vi "Write VISA Commands.vi"(6 "CMD Prefix":string, 7 "CMDs":string[](array[string]), 8 "error in":errorcluster, 9 "<JSON> Object":string, 10 "JSON Keys":string[](array[string]), 11 "VISA Refnum in":refnum<visa-resource-name>) -> (0 "error out":errorcluster, 3 "VISA Refnum out":refnum<visa-resource-name>)   [LabVIEW 2023, in "Continuous Waveform Acq CFG.lvclass"]
uses:
  Continuous Waveform Acq CFG.lvclass
  98ddc1df-d889-4f20-b281-f2799059f154.vi
  <vilib>/JDP Science/JSONtext/Find Item.vi
  <vilib>/JDP Science/JSONtext/Next JSON Value.vi
  <vilib>/JDP Science/JSONtext/String Subset.vi
  <vilib>/JDP Science/JSONtext/Parsing/Advance past next JSON Value (inlined COPY).vi
  <vilib>/JDP Science/JSONtext/Parsing/Advance past whitespace.vi
  <vilib>/JDP Science/JSONtext/Parsing/Advance past String.vi
  <vilib>/JDP Science/JSONtext/Parsing/Advance past Number.vi
  <vilib>/JDP Science/JSONtext/Parsing/Advance past Line Ending.vi
  <vilib>/JDP Science/JSONtext/Parsing/Parse Full Path or Item Name.vi
  <vilib>/JDP Science/JSONtext/Parsing/Advance past Array.vi
  <vilib>/JDP Science/JSONtext/Parsing/Advance past Object.vi
  <vilib>/JDP Science/JSONtext/support/Error Cluster From Code.vi
  <vilib>/JDP Science/JSONtext/Offset/Find Item Locations by Path.vi
  <vilib>/JDP Science/JSONtext/JSON text to Variant.vi
  <vilib>/ErrorRing/Error Ring.xnode
  <vilib>/JDP Science/JSONtext/LVClass Serializer/JSONtext LVClass Serializer.lvclass
  Continuous Waveform Acq CFG.lvclass/Continuous Waveform Acq CFG.ctl
  OWON SDS1022.lvclass
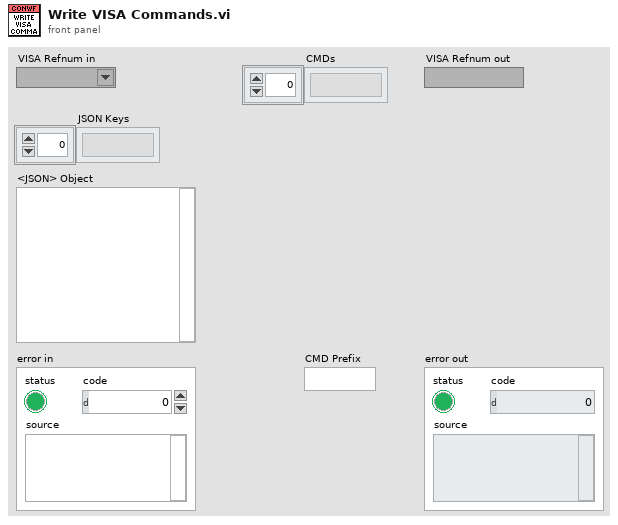
[diagram p1: front panel]
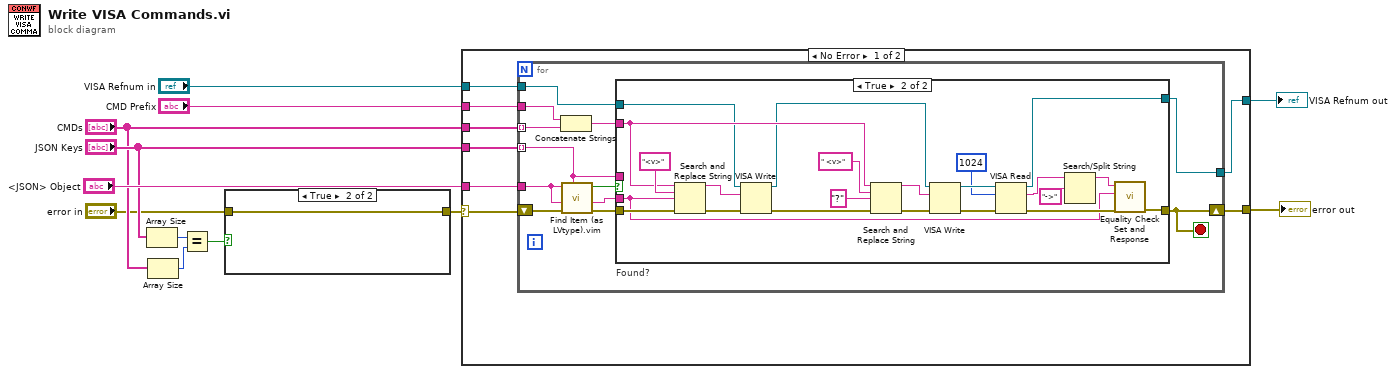
[diagram p0: block diagram]
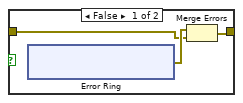
[diagram p2: hidden frame]
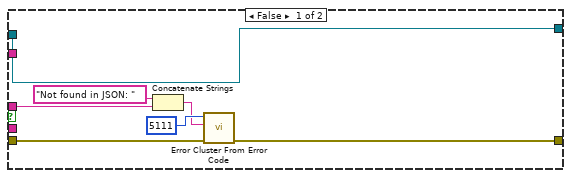
[diagram p3: hidden frame]
diagram:
  n1 = Array Size(array="JSON Keys") -> (size(s)=w4:i32)
  n2 = Array Size(array="CMDs") -> (size(s)=w5:i32)
  n3 = Equal?(x=w4, y=w5) -> (x = y?=w1:bool)
  n4 = case shown="True" w1 {
    tunnel: "error in" -> [w13 w21]
    tunnel: [w15 w21] -> w2
    frame False {
      n5 = xnode "Error Ring"() -> ("error out"=w14:errorcluster)
      n6 = Merge Errors(w14, w13) -> (w15:errorcluster)
    }
    frame True {
    }
  }
  n7 = case shown="No Error" w2 {
    selector: w2 -> [w24 w72]
    tunnel: "<JSON> Object" -> [w27 _]
    tunnel: "CMD Prefix" -> [w29 _]
    tunnel: "VISA Refnum in" -> [w28 w71]
    tunnel: "CMDs" -> [w26 _]
    tunnel: "JSON Keys" -> [w25 _]
    tunnel: [w22 w72] -> w9
    tunnel: [w23 w71] -> w8
    frame No Error {
      n8 = for {
        tunnel: w27 -> [w30]
        tunnel: w25 -> [w32] mode=indexing
        tunnel: w26 -> [w37] mode=indexing
        tunnel: w28 -> [w40]
        shift-right: [w33] -> w22
        shift-left: w24 -> [w41]
        tunnel: w29 -> [w38]
        tunnel: [w31] -> w23
        stop <- w33 stop-if-true
        n9 = Concatenate Strings(w38, w37) -> (w36:string)
        n10 = call "Find Item (as LVtype).vim"("$Path or Item Name"=w32, "error in (no error)"=w41, "Data Type and Default Value"=w30, "JSON"=w30) -> ("error out"=w39:errorcluster, "Data"=w35:string, "Found"=w34:bool)  [unwired: 4 in, 1 out]
        n11 = case "Found?" shown="True" w34 {
          tunnel: w40 -> [w42 w60]
          tunnel: w39 -> [w48 w70]
          tunnel: w36 -> [_ w63]
          tunnel: w35 -> [_ w49]
          tunnel: [w47 w51] -> w33
          tunnel: w32 -> [w44 _]
          tunnel: [w42 w56] -> w31
          frame False {
            n12 = Concatenate Strings("Not found in JSON: " ("string"), w44) -> (w45:string)
            n13 = call <vilib>:"Error Cluster From Error Code.vi"("error in (no error)"=w48, "error message (\"\")"=w45, "error code (0)"=5111) -> ("error out"=w47:errorcluster)  [unwired: 6 in]
          }
          frame True {
            n14 = Search and Replace String(input string=w63, search string="<v>", replace string=w49, error in=w70) -> (result string=w67:string, error out=w68:errorcluster)  [unwired: 4 in, 2 out]
            n15 = VISA Write(VISA resource name=w60, write buffer=w67, error in (no error)=w68) -> (VISA resource name out=w58:refnum<visa-resource-name>, error out=w66:errorcluster)  [unwired: 1 out]
            n16 = Search and Replace String(input string=w63, search string=" <v>", replace string="?" ("replace string (\"\")"), error in=w66) -> (result string=w59:string, error out=w64:errorcluster)  [unwired: 4 in, 2 out]
            n17 = VISA Write(VISA resource name=w58, write buffer=w59, error in (no error)=w64) -> (VISA resource name out=w57:refnum<visa-resource-name>, error out=w65:errorcluster)  [unwired: 1 out]
            n18 = VISA Read(VISA resource name=w57, byte count=u32 1024, error in (no error)=w65) -> (VISA resource name out=w56:refnum<visa-resource-name>, read buffer=w53:string, error out=w52:errorcluster)  [unwired: 1 out]
            n19 = Search/Split String(string=w53, search string/char (-)="->") -> (substring before match=w50:string)  [unwired: 1 in, 2 out]
            n20 = call "Equality Check Set and Response.vi"("error in (no error)"=w52, "Sent"=w49, "Response"=w50) -> ("error out"=w51:errorcluster)  [unwired: 8 in]
          }
        }
      }
    }
    frame Error {
    }
  }
  "error out" <- w9
  "VISA Refnum out" <- w8
